vi "nm.offset&mult.vi"(10 "DyeLaser":T1, 11 "Mono":T2) -> (2 "y multiplier (nm/pixel)":dbl, 3 "y offset (nm)":dbl)   [LabVIEW 2022 SP3]
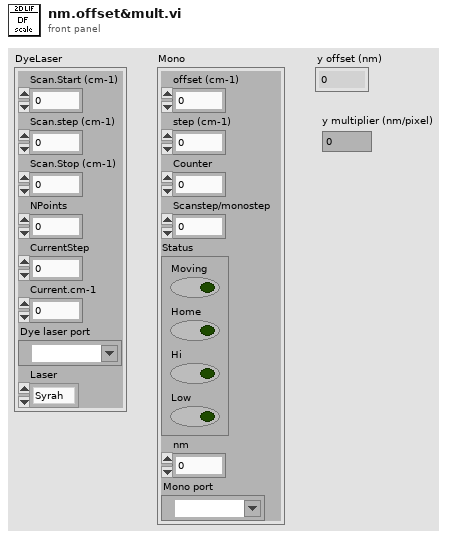
[diagram p1: front panel]
types:
  T1 = cluster{"Scan.Start (cm-1)":dbl, "Scan.Stop (cm-1)":dbl, "Scan.step (cm-1)":dbl, "Dye laser port":refnum<visa-resource-name>, "Laser":enum16{"Syrah", "Hyperdye"}, "NPoints":i32, "CurrentStep":i32, "Current.cm-1":dbl}
  T2 = cluster{"offset (cm-1)":dbl, "step (cm-1)":dbl, "Counter":dbl, "Scanstep/monostep":i32, "Status":cluster{"Moving":bool, "Home":bool, "Hi":bool, "Low":bool}, "nm":dbl, "Mono port":refnum<visa-resource-name>}
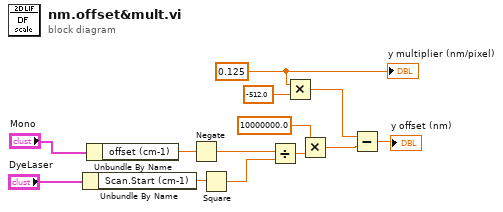
[diagram p0: block diagram]
diagram:
  w3 = 0.125
  n1 = Unbundle By Name("DyeLaser") -> ("Scan.Start (cm-1)"=w6:dbl)
  n2 = Unbundle By Name("Mono") -> ("offset (cm-1)"=w7:dbl)
  n3 = Negate(x=w7) -> (-x=w11:dbl)
  n4 = Square(x=w6) -> (x^2=w8:dbl)
  n5 = Divide(x=w11, y=w8) -> (x/y=w9:dbl)
  n6 = Multiply(x=w3, y=-512.0) -> (x*y=w1:dbl)
  n7 = Multiply(x=10000000.0, y=w9) -> (x*y=w12:dbl)
  n8 = Subtract(x=w1, y=w12) -> (x-y=→"y offset (nm)":dbl)
  "y multiplier (nm/pixel)" <- w3
